vi "CoboltLaser_ComPortRead.vi"(0 "ComPort":refnum<visa-resource-name>, 5 "error in (no error)":errorcluster) -> (14 "ComPort Out":refnum<visa-resource-name>, 15 "Response":string, 19 "error out":errorcluster)   [LabVIEW 2019]
doc: "Use this template to build a VI to use as a subVI."
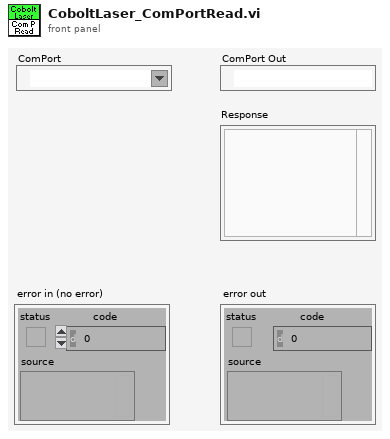
[diagram p1: front panel]
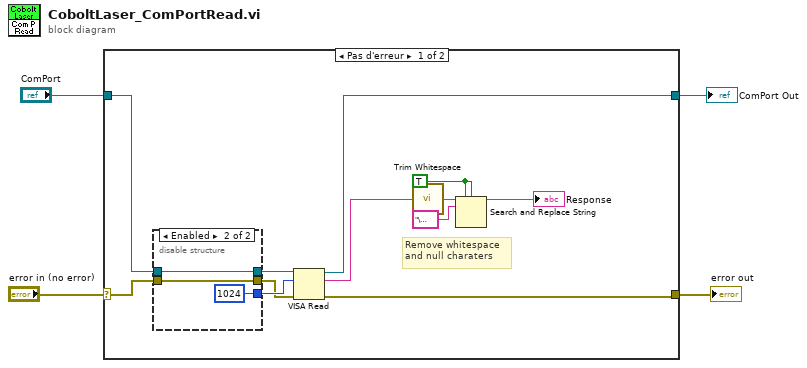
[diagram p0: block diagram]
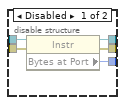
[diagram p2: hidden frame]
diagram:
  n1 = case shown="Pas d'erreur" "error in (no error)" {
    selector: "error in (no error)" -> [w12 w26]
    tunnel: [w13 w26] -> w3
    tunnel: "ComPort" -> [w6 w25]
    tunnel: [w5 w25] -> w1
    frame No Error {
      w9 = TRUE ("replace all? (F)")
      # "Remove whitespace\nand null charaters"
      n2 = disable-structure shown="Enabled" {
        disable-tunnel: [w21 w24] -> w16
        disable-tunnel: [w20 u32 1024 ("Bytes at Port")] -> w15
        disable-tunnel: [w19 w23] -> w14
        disable-tunnel: w12 -> [w18 w23]
        disable-tunnel: w6 -> [w17 w24]
        frame Disabled {
          n3 = property class="Instr"(reference=w17, error in=w18) -> (reference out=w21:refnum<visa-resource-name>, error out=w19:errorcluster, "Bytes at Port"=w20:u32)
        }
        frame Enabled {
        }
      }
      n4 = VISA Read(VISA resource name=w16, byte count=w15, error in (no error)=w14) -> (VISA resource name out=w5:refnum<visa-resource-name>, read buffer=w8:string, error out=w13:errorcluster)  [unwired: 1 out]
      n5 = call <vilib>:"Trim Whitespace.vi"("string"=w8) -> ("trimmed string"=w11:string)  [unwired: 1 in]
      n6 = Search and Replace String(replace all?=w9, case sensitive?=w9, input string=w11, search string="\u0000") -> (result string=→"Response":string)  [unwired: 4 in, 3 out]
    }
    frame Error {
    }
  }
  "error out" <- w3
  "ComPort Out" <- w1
